vi "14- Remove trailing space (SubVI).vi"(11 "iNPUT STRING":string) -> (3 "oUTPUT STRING":string)   [LabVIEW 2019]
panel:
  # "SUBVI TO REMOVE TRAILING SPACE"
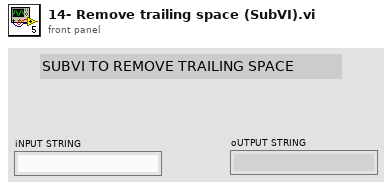
[diagram p1: front panel]
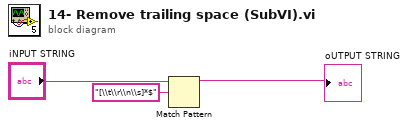
[diagram p0: block diagram]
diagram:
  n1 = Match Pattern(string="iNPUT STRING", regular expression="[\\t\\r\\n\\s]*$") -> (before substring=→"oUTPUT STRING":string)  [unwired: 1 in, 3 out]
